vi "libssh2_channel_process_startup.vi"(8 "error in (no error)":errorcluster, 9 "message":string, 10 "request":string, 11 "channel":u64) -> (0 "error out":errorcluster, 3 "return value":i32)   [LabVIEW 2013, in "libssh2.lvlib"]
uses:
  libssh2.lvlib
  libssh2.dll
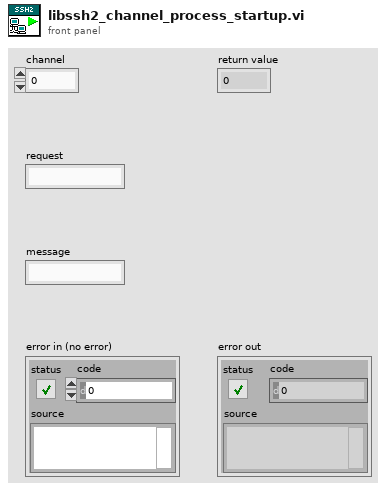
[diagram p1: front panel]
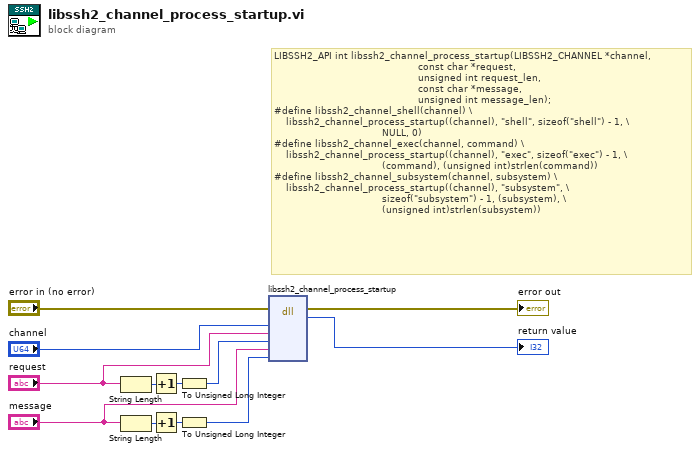
[diagram p0: block diagram]
diagram:
  # "LIBSSH2_API int libssh2_channel_process_startup(LIBSSH2_CHANNEL *channel,\n                                                const char *request,\n                                                unsigned int request_len,\n                                                const char *message,\n                                                unsigned int message_len);\n#define libssh2_channel_shell(channel) \\\n    libssh2_channel_process_startup((channel), \"shell\", sizeof(\"shell\") - 1, \\\n                                    NULL, 0)\n#define libssh2_channel_exec(channel, command) \\\n    libssh2_channel_process_startup((channel), \"exec\", sizeof(\"exec\") - 1, \\\n                                    (command), (unsigned int)strlen(command))\n#define libssh2_channel_subsystem(channel, subsystem) \\\n    libssh2_channel_process_startup((channel), \"subsystem\", \\\n                                    sizeof(\"subsystem\") - 1, (subsystem), \\\n                                    (unsigned int)strlen(subsystem))"
  n1 = String Length(string="request") -> (length=w12:i32)
  n2 = String Length(string="message") -> (length=w7:i32)
  n3 = Increment(x=w12) -> (x+1=w11:i32)
  n4 = Increment(x=w7) -> (x+1=w8:i32)
  n5 = To Unsigned Long Integer(number=w11) -> (unsigned 32bit integer=w9:u32)
  n6 = To Unsigned Long Integer(number=w8) -> (unsigned 32bit integer=w6:u32)
  n7 = dll-call lib="C:/Users/pasca/source/repos/libssh2-labview/libssh2**.*" fn="libssh2_channel_process_startup"(error in="error in (no error)", "channel"="channel", "request"="request", "request_len"=w9, "message"="message", "message_len"=w6) -> (error out=→"error out":errorcluster, "return value"=→"return value":i32)  [unwired: 7 in, 1 out]
